vi "Create reply queue bindings (SubVI).vi"(2 "error in (no error)":errorcluster, 3 "reply queue name":string, 4 "Exchange.lvclass":refnum<class "Exchange.lvclass">, 5 "Queue in":refnum<class "Queue.lvclass">) -> (0 "error out":errorcluster, 1 "Queue out":refnum<class "Queue.lvclass">)   [LabVIEW 2016]
uses:
  <vilib>/Distrio/LabbitMQ/Queue/Queue.lvclass
  <vilib>/Distrio/LabbitMQ/Exchange/Exchange.lvclass
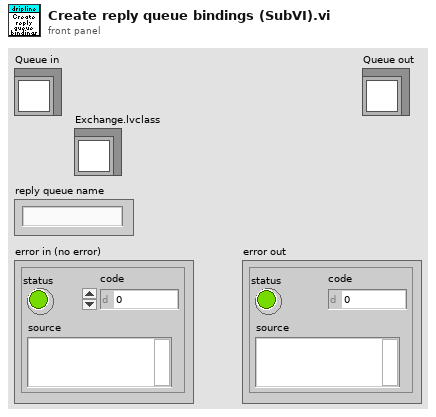
[diagram p1: front panel]
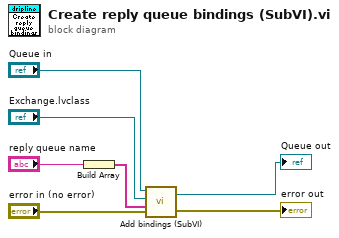
[diagram p0: block diagram]
diagram:
  n1 = Build Array("reply queue name") -> (w1:string[])
  n2 = call "Add bindings (SubVI).vi"("error in (no error)"="error in (no error)", "binding key"=w1, "Exchange.lvclass"="Exchange.lvclass", "Queue in"="Queue in") -> ("error out"=→"error out":errorcluster, "Queue out"=→"Queue out":refnum<class "Queue.lvclass">)
